vi "Synth Enter Serial Mode.vi"(8 "Error In":errorcluster, 11 "DAQmx Device Name":tag) -> (0 "Error Out":errorcluster, 3 "DAQmx Device Name out":tag)   [LabVIEW 2021]
uses:
  <vilib>/DAQmx/write.llb/DAQmx Write (Digital 1D Bool 1Chan 1Samp).vi
  <vilib>/DAQmx/create/channels.llb/DAQmx Create Channel (DO-Digital Output).vi
  <vilib>/DAQmx/miscellaneous.llb/DAQmx Fill In Error Info.vi
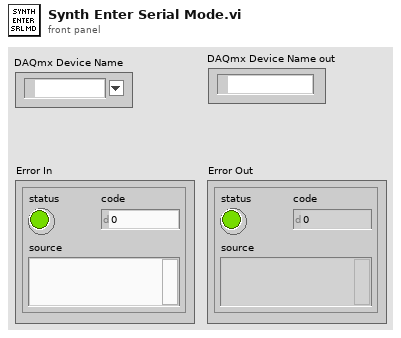
[diagram p1: front panel]
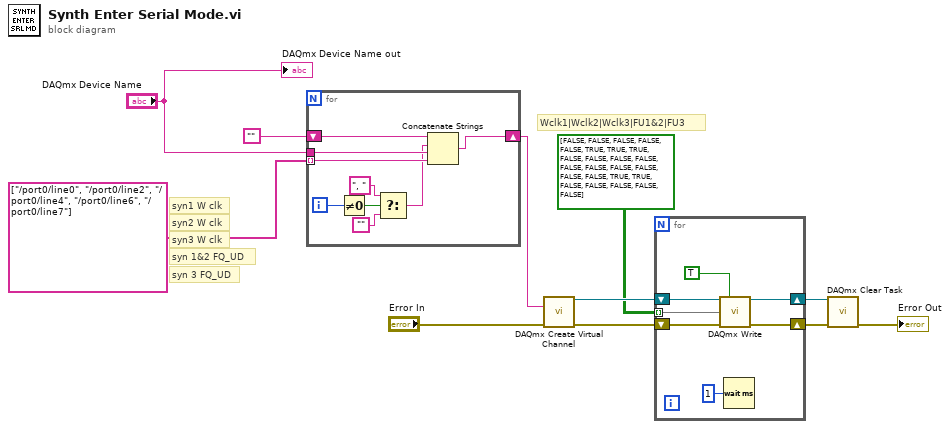
[diagram p0: block diagram]
diagram:
  # "syn 3 FQ_UD"
  # "syn 1&2 FQ_UD"
  # "syn3 W clk"
  # "syn2 W clk"
  # "syn1 W clk"
  # "Wclk1|Wclk2|Wclk3|FU1&2|FU3"
  n1 = for {
    shift-right: [w17] -> w4
    shift-left: "" -> [w18]
    tunnel: "DAQmx Device Name" -> [w20]
    tunnel: string[] ["/port0/line0", "/port0/line2", "/port0/line4", "/port0/line6", "/port0/line7"] -> [w19] mode=indexing
    i -> [w16]
    n2 = Not Equal To 0?(x=w16) -> (x != 0?=w15:bool)
    n3 = Select(t=", ", s=w15, f="") -> (s? t:f=w12:string)
    n4 = Concatenate Strings(w18, w12, w20, w19) -> (w17:string)
  }
  n5 = call-poly <vilib>:"DAQmx Create Virtual Channel.vi"("lines"=w4, "error in"="Error In") -> ("task out"=w10:refnum<k21>, "error out"=w11:errorcluster)  [unwired: 3 in, 9 out]
  n6 = for {
    shift-right: [w25] -> w9
    shift-left: w11 -> [w27]
    shift-right: [w24] -> w8
    shift-left: w10 -> [w26]
    tunnel: bool[][] [[FALSE, FALSE, FALSE, FALSE, FALSE], [TRUE, TRUE, TRUE, FALSE, FALSE], [FALSE, FALSE, FALSE, FALSE, FALSE], [FALSE, FALSE, FALSE, TRUE, TRUE], [FALSE, FALSE, FALSE, FALSE, FALSE]] -> [w21] mode=indexing
    n7 = call-poly <vilib>:"DAQmx Write.vi"("task/channels in"=w26, "auto start"=TRUE, "data"=w21, "error in"=w27) -> ("task out"=w24:refnum<k21>, "error out"=w25:errorcluster)  [unwired: 10 out]
    n8 = Wait (ms)(milliseconds to wait=u32 1) -> ()  [unwired: 1 out]
  }
  n9 = call <vilib>:"DAQmx Clear Task.vi"("task in"=w8, "error in"=w9) -> ("error out"=→"Error Out":errorcluster)  [unwired: 13 out]
  "DAQmx Device Name out" <- "DAQmx Device Name"
